vi "Read lockin configuration  DDS.vi"(0 "tdms file":refnum<k34>, 1 "Pipeline delay":dbl=28.0, 5 "group name in":string, 9 "Channel name":string, 11 "Error In":errorcluster, 12 "Sample rate":dbl=125000000.0 format="%#_6p", 13 "DDS phase modulus":u64=100000000 format="%x") -> (2 "dt":dbl, 3 "Frequency word":u32, 4 "tdms file out":refnum<k34>, 6 "Frequency":dbl format="%_19p", 8 "t0":timestamp, 10 "Phase":dbl, 14 "Phase word":u32, 15 "Error Out":errorcluster)   [LabVIEW 2016]
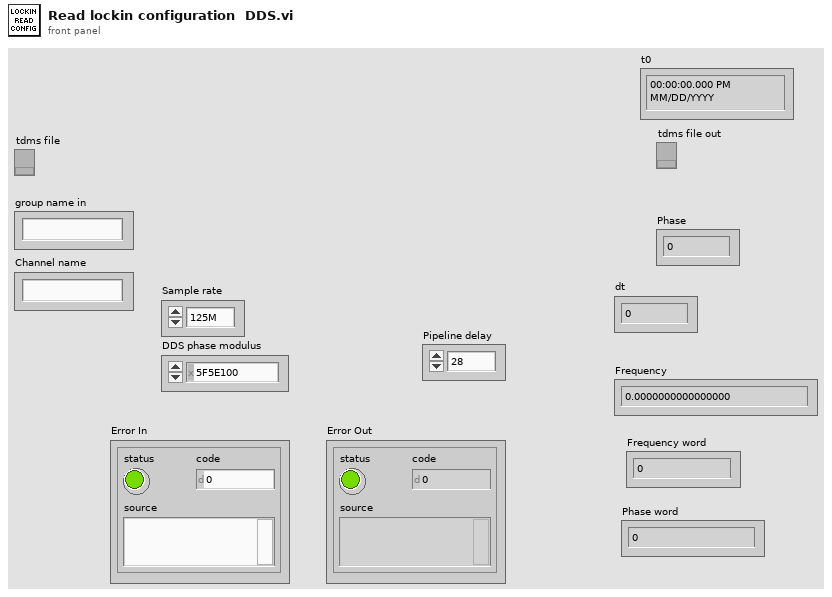
[diagram p1: front panel]
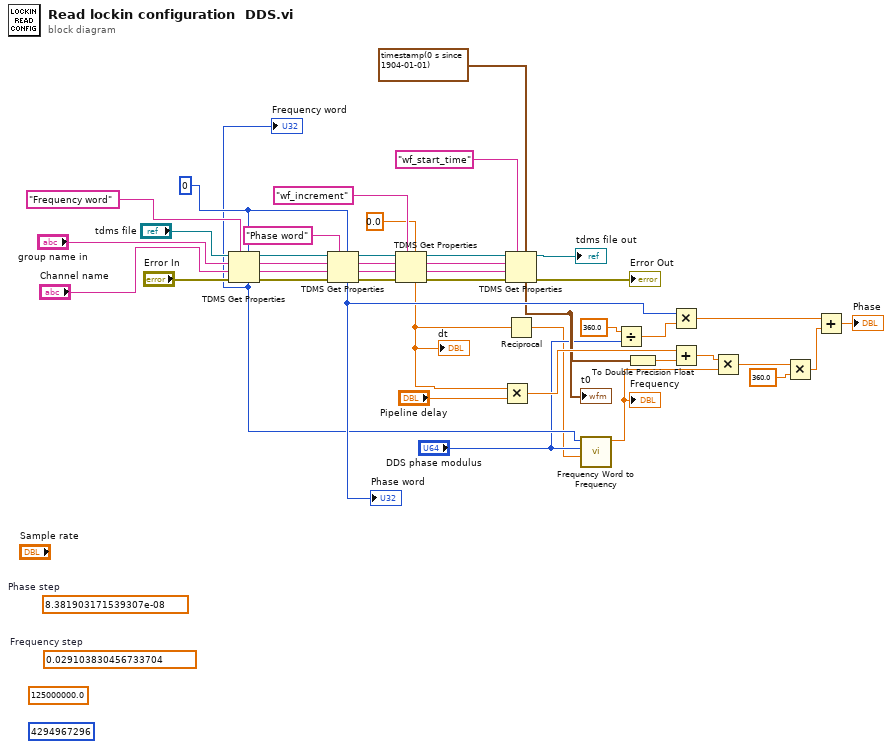
[diagram p0: block diagram]
diagram:
  w22 = u32 0 ("index")
  (unwired) 8.381903171539307e-08  # Phase step
  (unwired) 0.029103830456733704  # Frequency step
  (unwired) u64 4294967296
  (unwired) 125000000.0
  n1 = TDMS Get Properties(5:w22, 7:"Frequency word" ("name"), 8:"Error In", 9:"Channel name", 10:"group name in", 11:"tdms file") -> (0:w24:errorcluster, 1:w26:string, 2:w27:string, 3:w25:refnum<k34>, 4:w4:u32)  [unwired: 1 out]
  "Frequency word" <- w4
  n2 = TDMS Get Properties(5:w22, 7:"Phase word" ("name"), 8:w24, 9:w26, 10:w27, 11:w25) -> (0:w16:errorcluster, 1:w17:string, 2:w18:string, 3:w15:refnum<k34>, 4:w21:u32)  [unwired: 1 out]
  "Phase word" <- w21
  n3 = TDMS Get Properties(5:0.0, 7:"wf_increment", 8:w16, 9:w17, 10:w18, 11:w15) -> (0:w14:errorcluster, 1:w11:string, 2:w12:string, 3:w13:refnum<k34>, 4:w5:dbl)  [unwired: 1 out]
  "dt" <- w5
  n4 = Multiply(x=w5, y="Pipeline delay") -> (x*y=w38:dbl)
  n5 = TDMS Get Properties(5:timestamp(0 s since 1904-01-01) ("t0"), 7:"wf_start_time", 8:w14, 9:w11, 10:w12, 11:w13) -> (0:→"Error Out":errorcluster, 3:→"tdms file out":refnum<k34>, 4:w6:timestamp)  [unwired: 3 out]
  "t0" <- w6
  n6 = Reciprocal(x=w5) -> (1/x=w2:dbl)
  n7 = call "Frequency Word to Frequency .vi"("DDS clock"=w2, "DDS modulus"="DDS phase modulus", "Frequency word"=w4) -> ("Frequency"=w1:dbl)  [unwired: 8 in]
  "Frequency" <- w1
  n8 = Divide(x=360.0, y="DDS phase modulus") -> (x/y=w29:dbl)
  n9 = To Double Precision Float(number=w6) -> (double precision float=w43:dbl)
  n10 = Multiply(x=w21, y=w29) -> (x*y=w34:dbl)
  n11 = Add(x=w38, y=w43) -> (x+y=w39:dbl)
  n12 = Multiply(x=w39, y=w1) -> (x*y=w42:dbl)
  n13 = Multiply(x=w42, y=360.0) -> (x*y=w35:dbl)
  n14 = Add(x=w34, y=w35) -> (x+y=→"Phase":dbl)
